vi "PM5000_AlarmLog.vi"(8 "error in":errorcluster, 11 "Network Path":string="172.22.26.202") -> (0 "error out":errorcluster, 2 "Alarm Log":i16[](array[numeric]), 3 "Network Path out":string="192.168.169.1")   [LabVIEW 2018]
doc: "Lee la tabla de memoria RealTime_VIF_Power del equipo PowerMonitor 5000, ademas filtra y ordena las variables de interez de la tabla de memoria.\n\nLee las siguientes variables de la tabla RealTime_VIF_Power:\n\n*V1_V2_Volts\n*V2_V3_Volts\n*V3_V1_Volts\n*I1_Amps\n*I2_Amps\n*I3_Amps\n*Frequency_Hz\n*Total_kW\n*Total_kVAR\n*Total_kVA\n*Total_True_PF\n*Total_Disp_PF"
uses:
  <vilib>/ethernetip/ethernetip.llb/EthernetIP SLC500 Read Integer.vi
  <vilib>/ethernetip/ethernetip.lvlib
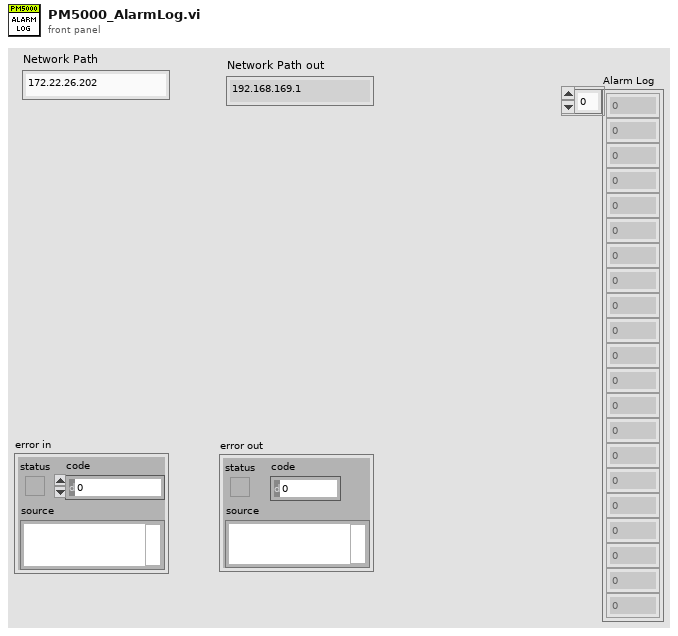
[diagram p1: front panel]
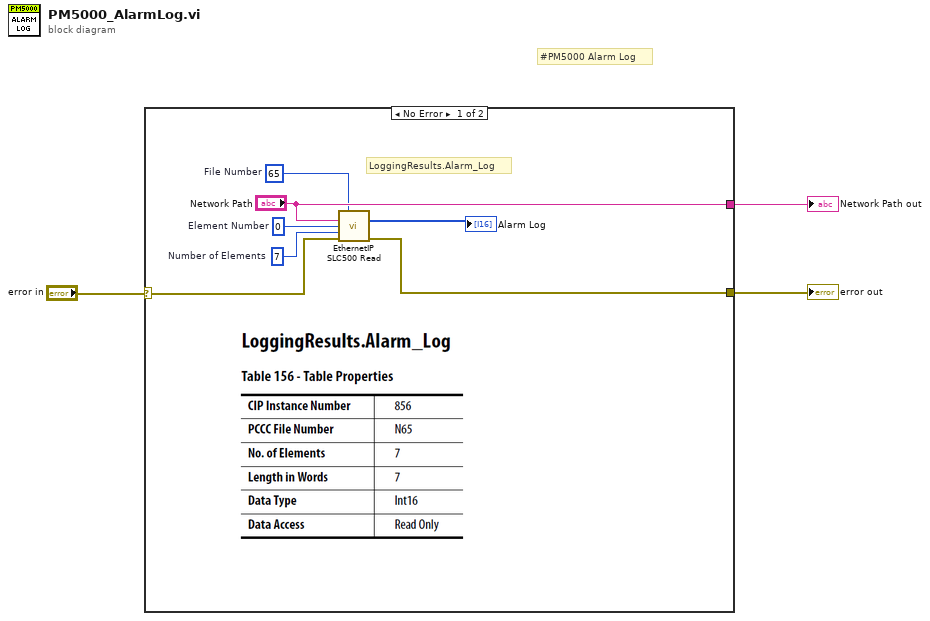
[diagram p0: block diagram]
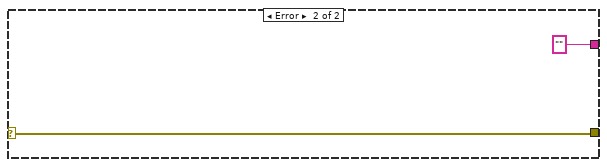
[diagram p2: hidden frame]
diagram:
  # "#PM5000 Alarm Log"
  n1 = case shown="No Error" "error in" {
    selector: "error in" -> [w5 w11]
    tunnel: [w10 w11] -> w3
    tunnel: ["Network Path" "" ("Network Path")] -> w2
    frame No Error {
      w6 = u32 7  # Number of Elements
      w8 = u16 65  # File Number
      w7 = u16 0  # Element Number
      # "LoggingResults.Alarm_Log"
      n2 = call-poly <vilib>:"EthernetIP SLC500 Read.vi"("File Number"=w8, "Network Path"="Network Path", "Element Number"=w7, "Number of Elements"=w6, "error in"=w5) -> ("Data"=→"Alarm Log":i16[], "error out"=w10:errorcluster)  [unwired: 8 in, 1 out]
    }
    frame Error {
    }
  }
  "error out" <- w3
  "Network Path out" <- w2
